vi "GEOM_VAR_CoordsRef.vi"(9 "Action":T2, 10 "GEOM_coordsref":T1) -> (2 "GEOM_coordsref out":T1)   [LabVIEW 2016]
uses:
  GEOM_VAR_action.ctl
  GEOM_CoordsRef.ctl
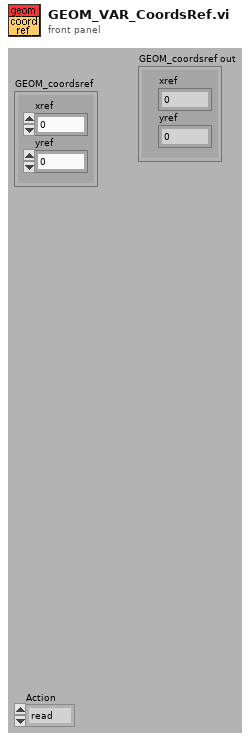
[diagram p1: front panel]
types:
  T1 = typedef "GEOM_CoordsRef.ctl" = cluster{"xref":u32, "yref":u32}
  T2 = typedef "GEOM_VAR_action.ctl" = enum16{"read", "write"}
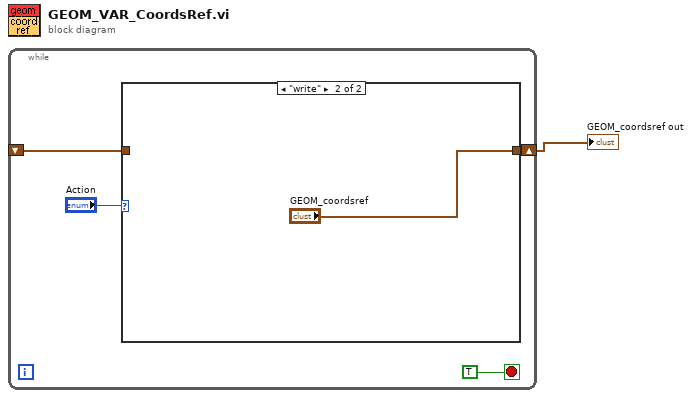
[diagram p0: block diagram]
diagram:
  n1 = while {
    shift-right: [w2] -> w1
    shift-left: _ -> [w4]
    stop <- TRUE stop-if-true
    n2 = case shown="\"write\"" "Action" {
      tunnel: w4 -> [w6 _]
      tunnel: [w6 "GEOM_coordsref"] -> w2
      frame "read", Default {
      }
      frame "write" {
      }
    }
  }
  "GEOM_coordsref out" <- w1
